vi "SHA-512-224 Byte Array Checksum.vi"(11 "buffer":u8[](array[numeric]) format="%02x") -> (3 "digest":string)   [LabVIEW 2020, in "NI_Message Digest API.lvlib"]
doc: "Computes the message digest on a byte array. You must manually select the polymorphic instance you want to use."
uses:
  <vilib>/security/Message Digest/API/NI_Message Digest API.lvlib
  6b0a94b4-5f98-45be-8858-b3dd3cac734b.vi
  6b0a94b4-5f98-45be-8858-b3dd3cac734b.vi/8d2e9b66-293e-3fec-60db-660b807ccc3f.vi
  <vilib>/security/Message Digest/SHA-2/SHA-512/Get Block Size.vi
  <vilib>/security/Message Digest/SHA-2/SHA-512/Reset.vi
  <vilib>/security/Message Digest/SHA-2/SHA-512/Append Block.vi
  <vilib>/security/Message Digest/SHA-2/SHA-512/Pad.vi
  <vilib>/security/Message Digest/SHA-2/SHA-512/Get Digest.vi
  <vilib>/security/Message Digest/SHA-2/SHA-512/NI_SHA-512.lvclass
  <vilib>/Bit Manipulation/NI_Bit Manipulation.lvlib
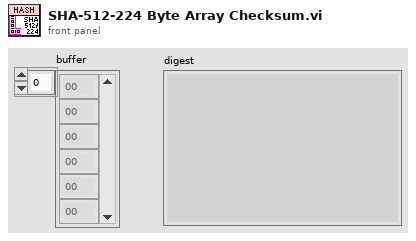
[diagram p1: front panel]
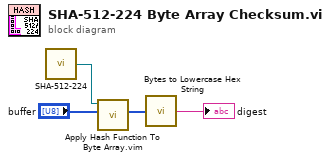
[diagram p0: block diagram]
diagram:
  n1 = call <vilib>:"SHA-512-224.vi"() -> ("Hash Function out"=w3:refnum<class "NI_SHA-512.lvclass">)
  n2 = call "Apply Hash Function To Byte Array.vim"("buffer"="buffer", "Hash Function in (SHA-256)"=w3) -> ("digest"=w1:u8[])  [unwired: 8 in, 1 out]
  n3 = call <vilib>:"Bytes to Lowercase Hex String.vi"("bytes"=w1) -> ("hex string"=→"digest":string)
